vi "L1OC_Phase_computation.vi"() -> (6 "Массив индексов фазы кода":i32[](array[numeric]))   [LabVIEW 2020]
uses:
  <vilib>/Analysis/2dsp.llb/Complex FFT.vi
  <vilib>/measure/maspectr.llb/FFT Power Spectrum and PSD for 1 Chan (CDB).vi
  <vilib>/Analysis/NI_AALPro.lvlib
  <vilib>/measure/NI_MAPro.lvlib
  <vilib>/Analysis/NI_AALBase.lvlib
panel:
  out "size(s)":i32
  out "size(s) 2":i32
  out "Numeric":i32
  in  "file path (use dialog)":path=path "C:/Users/ira_1/OneDrive/Рабочий стол/samples.bin"
  in  "qc/N0":dbl=50.0
  out "Waveform Graph 3":cluster{"f0":dbl, "df":dbl, "magnitude":dbl[]}(graph)
  out "Waveform Graph 2":waveform(dbl)(graph)
  in  "stop":bool
  in  "Частота\n дикретизации, Гц":dbl=5000000.0
  in  "Доплер\nнесущей, Гц":dbl=1000.0
  in  "Несущая\nчастота, Гц":dbl=1575450000.0
  in  "Задержка\nкода, симв":dbl=1.0
  out "Waveform Graph":dbl[](graph)
  out "Array":cdb[](array[numeric])
  out "доплер нес":dbl
  out "доплер код":dbl
  out "index of element":i32
  # "Блок вычисления фазы кода для составного сигнала КА"
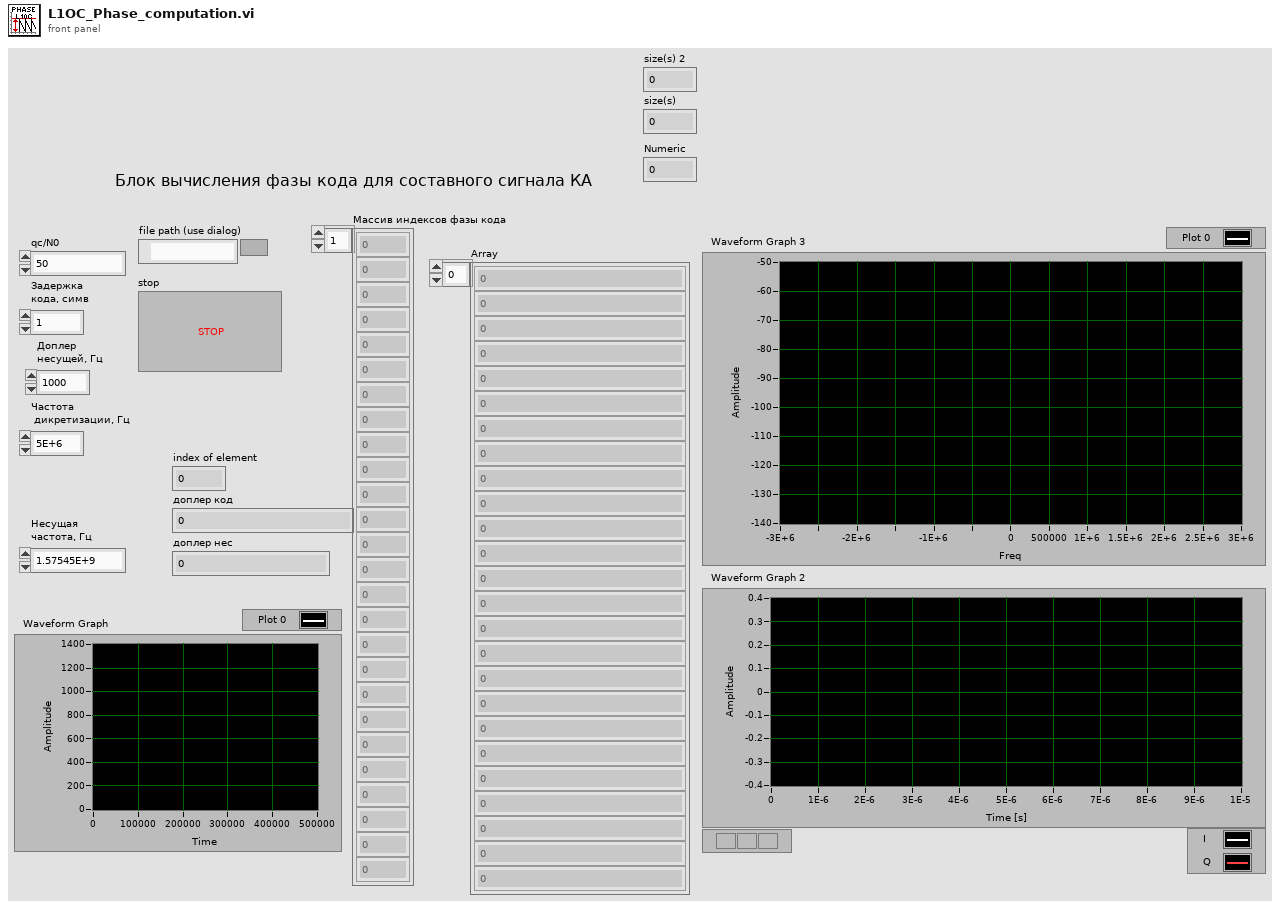
[diagram p1: front panel]
types:
  T1 = enum16{"open", "replace", "create", "open or create", "replace or create", "replace or create with confirmation"}
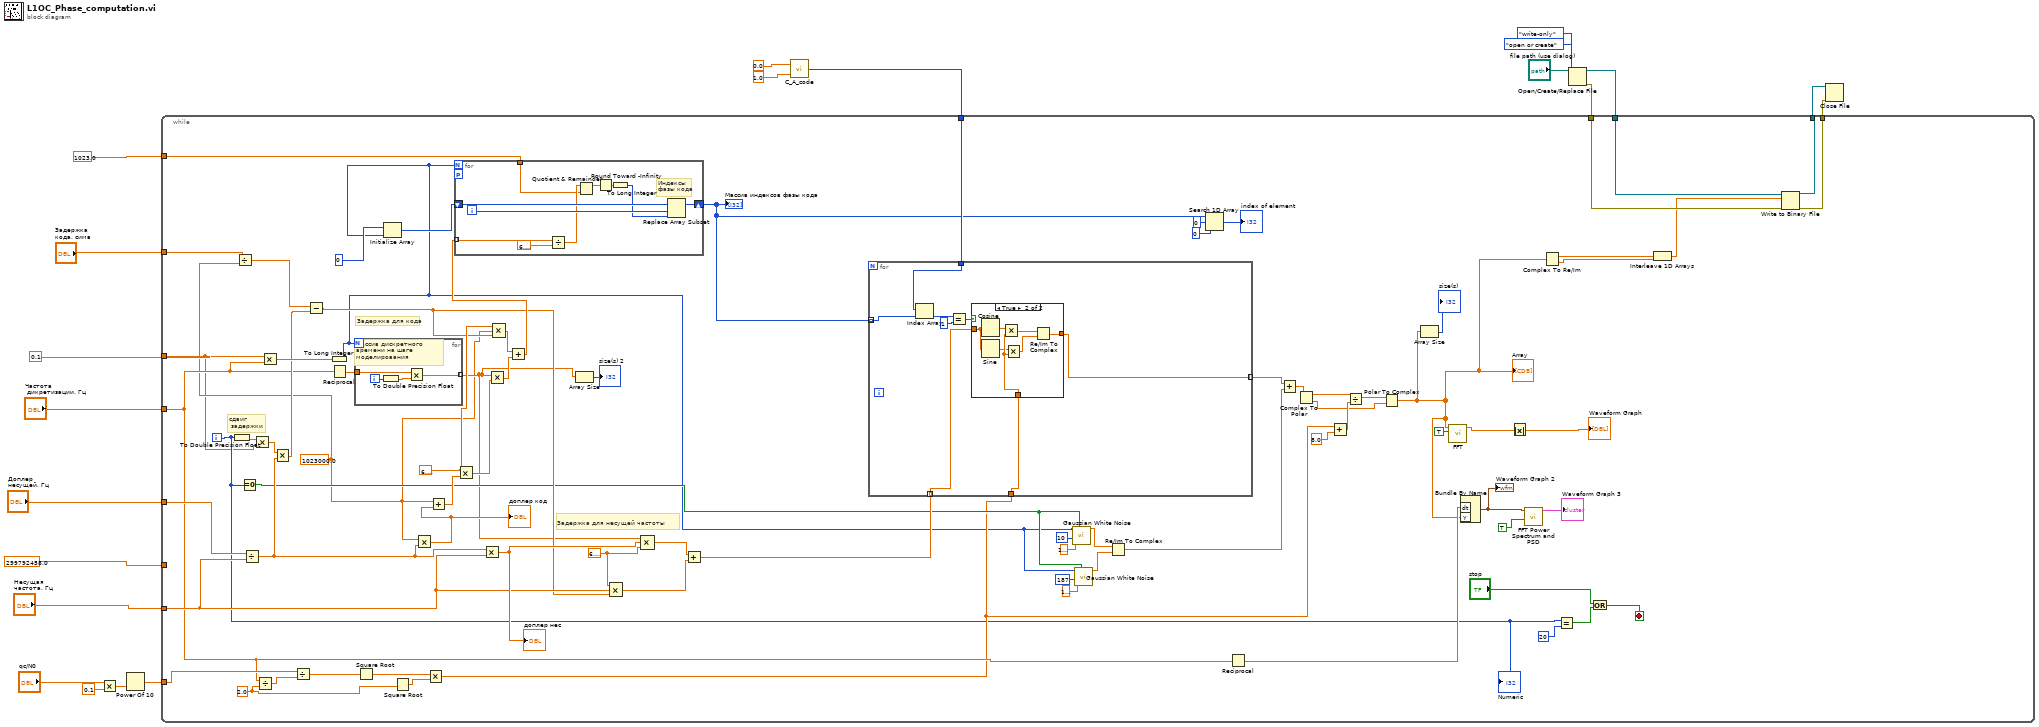
[diagram p0: block diagram]
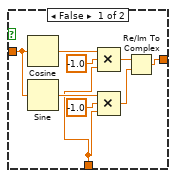
[diagram p2: hidden frame]
diagram:
  n1 = Multiply(x="qc/N0", y=0.1) -> (x*y=w10:dbl)
  n2 = Power Of 10(x=w10) -> (10^x=w9:dbl)
  n3 = call "C_A_code.vi"("NKA id"=1.0, "Delay"=0.0) -> ("Value"=w18:i32[])
  n4 = Open/Create/Replace File(file path (use dialog)="file path (use dialog)", operation (0:open)=T1."open or create", access (0:read/write)=enum16{"read/write", "read-only", "write-only"}."write-only") -> (refnum out=w7:refnum<file>, error out=w4:errorcluster)  [unwired: 3 in, 1 out]
  n5 = while {
    tunnel: 0.1 ("x") -> [w24]
    tunnel: w18 -> [w91]
    tunnel: "Задержка\nкода, симв" -> [w78]
    tunnel: "Доплер\nнесущей, Гц" -> [w75]
    tunnel: 299792458.0 ("y") -> [_]
    tunnel: "Несущая\nчастота, Гц" -> [w70]
    tunnel: "Частота\n дикретизации, Гц" -> [w55]
    tunnel: w9 -> [w64]
    tunnel: w7 -> [w38]
    tunnel: w4 -> [w37]
    tunnel: [w36] -> w3
    tunnel: [w35] -> w2
    tunnel: 1023.0 -> [w23]
    i -> [w31]
    stop <- w39 stop-if-true
    w30 = 2.0
    w80 = 6.283185307179586
    w25 = 1023000.0 ("value")
    w99 = 6.283185307179586
    # "сдвиг\n задержки"
    # "Задержка для кода"
    # "Задержка для несущей частоты"
    n6 = To Double Precision Float(number=w31) -> (double precision float=w77:dbl)
    n7 = Divide(x=w78, y=w25) -> (x/y=w65:dbl)
    n8 = Equal To 0?(x=w31) -> (x = 0?=w58:bool)
    n9 = Divide(x=w75, y=w70) -> (x/y=w74:dbl)
    n10 = Multiply(x=w77, y=w24) -> (x*y=w76:dbl)
    n11 = Divide(x=w55, y=w30) -> (x/y=w54:dbl)
    n12 = Multiply(x=w24, y=w55) -> (x*y=w101:dbl)
    n13 = Multiply(x=w76, y=w74) -> (x*y=w66:dbl)
    n14 = Divide(x=w64, y=w54) -> (x/y=w63:dbl)
    n15 = Subtract(x=w65, y=w66) -> (x-y=w67:dbl)
    n16 = To Long Integer(number=w101) -> (32bit integer=w26:i32)
    n17 = Reciprocal(x=w55) -> (1/x=w100:dbl)
    n18 = for {
      N: w26 -> [_]
      tunnel: w100 -> [w127]
      tunnel: [w126] -> w28 mode=indexing
      i -> [w129]
      # "массив дискретного \nвремени на шаге \nмоделирования"
      n19 = To Double Precision Float(number=w129) -> (double precision float=w128:dbl)
      n20 = Multiply(x=w127, y=w128) -> (x*y=w126:dbl)
    }
    n21 = Square Root(x=w63) -> (sqrt(x)=w62:dbl)
    n22 = Initialize Array(0, w26) -> (w92:i32[])
    n23 = Square Root(x=w30) -> (sqrt(x)=w61:dbl)
    n24 = Multiply(x=w25, y=w74) -> (x*y=w68:dbl)
    "доплер код" <- w68
    n25 = Multiply(x=w62, y=w61) -> (x*y=w49:dbl)
    n26 = Add(x=w25, y=w68) -> (x+y=w98:dbl)
    n27 = Multiply(x=w99, y=w98) -> (x*y=w97:dbl)
    n28 = Multiply(x=w74, y=w70) -> (x*y=w79:dbl)
    "доплер нес" <- w79
    n29 = Multiply(x=w28, y=w97) -> (x*y=w96:dbl[])
    n30 = Compound Arithmetic op=MULTIPLY(w99, w25, w67) -> (w95:dbl)
    n31 = Add(x=w95, y=w96) -> (x+y=w94:dbl[])
    n32 = for {
      N: w26 -> [_]
      shift-right: [w137] -> w90
      shift-left: w92 -> [w136]
      workers-P: _ -> [_]
      tunnel: w94 -> [w133] mode=indexing
      tunnel: w23 -> [w130]
      i -> [w135]
      # "Индексы\nфазы кода"
      n33 = Divide(x=w133, y=6.283185307179586) -> (x/y=w131:dbl)
      n34 = Quotient & Remainder(x=w131, y=w130) -> (x-y*floor(x/y)=w138:dbl)  [unwired: 1 out]
      n35 = Round Toward -Infinity(1:w138) -> (0:w139:dbl)
      n36 = To Long Integer(number=w139) -> (32bit integer=w134:i32)
      n37 = Replace Array Subset(array=w136, new element=w134, index=w135) -> (w137:i32[])
    }
    "Массив индексов фазы кода" <- w90
    n38 = Array Size(array=w28) -> (size(s)=→"size(s) 2":i32)
    n39 = Compound Arithmetic op=MULTIPLY(w80, w70, w67) -> (w86:dbl)
    n40 = Compound Arithmetic op=MULTIPLY(w28, w79, w80) -> (w81:dbl[])
    n41 = Add(x=w81, y=w86) -> (x+y=w85:dbl[])
    n42 = for {
      tunnel: w91 -> [w109]
      tunnel: w90 -> [w108] mode=indexing
      tunnel: w85 -> [w104] mode=indexing
      tunnel: [w103] -> w50 mode=indexing
      tunnel: w49 -> [w102]
      n43 = Index Array(array=w109, index=w108) -> (element=w107:i32)
      n44 = Equal?(x=w107, y=1) -> (x = y?=w105:bool)
      n45 = case shown="True" w105 {
        tunnel: w104 -> [w118 w125]
        tunnel: [w117 w124] -> w103
        tunnel: w102 -> [w112 w121]
        frame False {
          n46 = Cosine(x=w118) -> (cos(x)=w115:dbl)
          n47 = Sine(x=w118) -> (sin(x)=w113:dbl)
          n48 = Compound Arithmetic op=MULTIPLY(w115, -1.0 ("y"), w112) -> (w110:dbl)
          n49 = Compound Arithmetic op=MULTIPLY(w113, -1.0 ("y"), w112) -> (w111:dbl)
          n50 = Re/Im To Complex(1:w111, 2:w110) -> (0:w117:cdb)
        }
        frame True {
          n51 = Cosine(x=w125) -> (cos(x)=w123:dbl)
          n52 = Sine(x=w125) -> (sin(x)=w120:dbl)
          n53 = Multiply(x=w123, y=w121) -> (x*y=w122:dbl)
          n54 = Multiply(x=w120, y=w121) -> (x*y=w119:dbl)
          n55 = Re/Im To Complex(1:w119, 2:w122) -> (0:w124:cdb)
        }
      }
    }
    n56 = call <vilib>:"Gaussian White Noise.vi"("initialize?"=w58, "seed"=10, "standard deviation"=1.0000000000000002, "samples"=w26) -> ("Gaussian noise pattern"=w53:dbl[])  [unwired: 6 in, 1 out]
    n57 = call <vilib>:"Gaussian White Noise.vi"("initialize?"=w58, "seed"=187, "standard deviation"=1.0000000000000002, "samples"=w26) -> ("Gaussian noise pattern"=w52:dbl[])  [unwired: 6 in, 1 out]
    n58 = Re/Im To Complex(1:w52, 2:w53) -> (0:w51:cdb[])
    n59 = Search 1D Array(1D array=w90, element=0, start index (0)=0) -> (index of element=→"index of element":i32)
    n60 = Reciprocal(x=w55) -> (1/x=w69:dbl)
    n61 = Add(x=w50, y=w51) -> (x+y=w47:cdb[])
    n62 = Complex To Polar(r * e^(i*theta)=w47) -> (r=w46:dbl[], theta=w43:dbl[])
    n63 = Add(x=w49, y=8.0) -> (x+y=w45:dbl)
    n64 = Divide(x=w46, y=w45) -> (x/y=w44:dbl[])
    n65 = Polar To Complex(1:w43, 2:w44) -> (0:w29:cdb[])
    "Array" <- w29
    n66 = Array Size(array=w29) -> (size(s)=→"size(s)":i32)
    n67 = call-poly <vilib>:"FFT.vi"("shift?"=TRUE, "X"=w29) -> ("FFT {X}"=w83:cdb[])  [unwired: 8 in, 1 out]
    n68 = Bundle By Name("dt"=w69, "Y"=w29) -> (w71:waveform(cdb))  [unwired: 1 in]
    "Waveform Graph 2" <- w71
    n69 = Absolute Value(x=w83) -> (abs(x)=→"Waveform Graph":dbl[])
    n70 = call-poly <vilib>:"FFT Power Spectrum and PSD.vi"("dB On (F)"=TRUE, "time signal"=w71) -> ("Power Spectrum / PSD"=→"Waveform Graph 3":cluster{"f0":dbl, "df":dbl, "magnitude":dbl[]})  [unwired: 6 in, 3 out]
    n71 = Complex To Re/Im(x + iy=w29) -> (x=w34:dbl[], y=w33:dbl[])
    n72 = Equal?(x=w31, y=20) -> (x = y?=w40:bool)
    n73 = Or(x="stop", y=w40) -> (x .or. y?=w39:bool)
    n74 = Interleave 1D Arrays(w34, w33) -> (w32:dbl[])
    n75 = Write to Binary File(file (use dialog)=w38, data=w32, error in=w37) -> (refnum out=w36:refnum<file>, error out=w35:errorcluster)  [unwired: 3 in, 1 out]
    "Numeric" <- w31
  }
  n76 = Close File(refnum=w3, error in=w2) -> ()  [unwired: 2 out]
